vi "Receptor.vi"() -> ()   [LabVIEW 2012]
uses:
  VariavelGlobalTDD.vi
panel:
  out "x = y?":bool caption="Se TDD on > Teste Passou?"
  in  "Boolean":bool caption="TDD"
  in  "stop 2":bool
  out "Dado Recebido:":string
  # "Rodar este VI antes de rodar Emissor.vi."
  # "1- Escolher TDD on ou off no switch;\n2- Rodar este VI;"
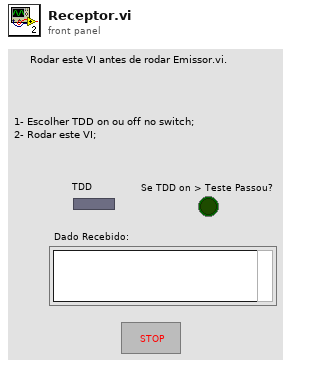
[diagram p1: front panel]
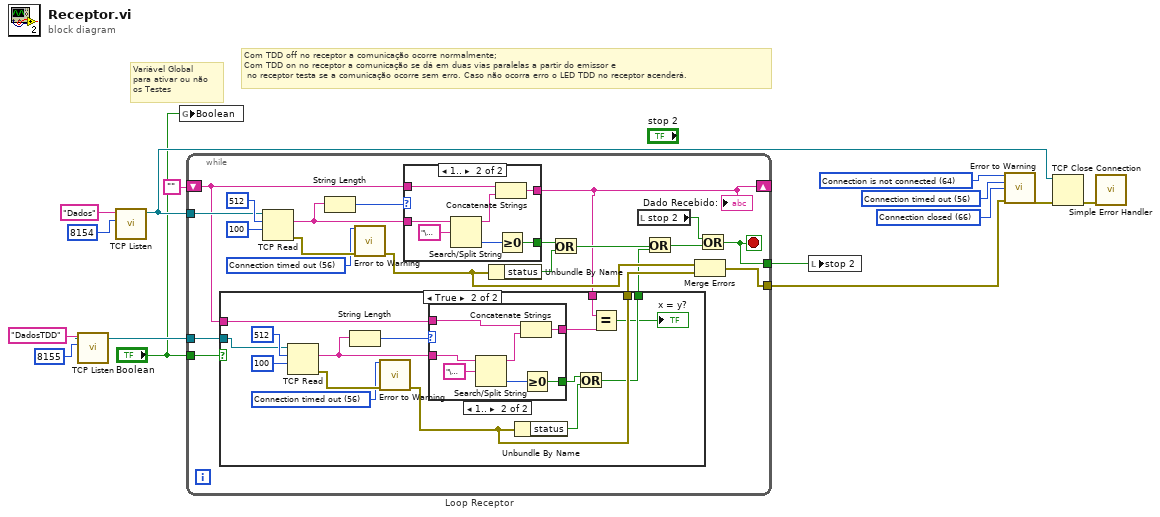
[diagram p0: block diagram]
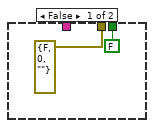
[diagram p2: hidden frame]
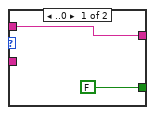
[diagram p3: hidden frame]
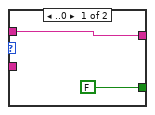
[diagram p4: hidden frame]
diagram:
  w8 = 56 items=["No Error", "Argument Error", "Memory Full", "Out of Zone", "End of File", "File Already Open", "Generic File IO Error", "File Not Found", "File Permission Error", "Disk Full", "Duplicate Path", "Too Many Files Open", "Not Enabled", "Resource File Not Found", "Cannot Add Resource", "Resource Not Found", "Image Not Found", "Image Memory Error", "Pen Does Not Exist", "Config Bad Type", "Config Token Not Found", "Config Parse Error", "Config Memory Error", "Bad External Code Format", "Bad External Code Offset", "External Code Not Present", "Null Window", "Destroy Window Mixup", "Null Menu", "Print Aborted", "Bad Print Record", "Print Driver Error", "Windows Error During Print", "Memory Error During Print", "Print Dialog Error", "Generic Print Error", "Invalid Device Refnum", "Device Not Found", "Device Parameter Error", "Device Unit Error", "Can't Open Device", "Device Call Aborted", "Generic Error", "Cancelled By User", "Object ID Too Low", "Object ID Too High", "Object Not In Heap", "Unknown Heap", "Bad DefProc ID", "DefProc Not In Table", "Message Out Of Range", "Null Method", "Unknown Message", "Manager Call Not Supported", "Bad address", "Connection In progress", "Connection timed out", "Connection is already in progress", "Network attribute not supported", "Network error", "Address in use", "System out of memory", "Connection aborted", "Connection refused", "Connection is not connected", "Connection is already connected", "Connection closed", "Initialize error (interapplication manager)", "Bad occurrence", "Wait on unbound occurrence handler", "Occurrence queue overflow", "Bad path", "Semaphore not signaled", "Unrecognized type (interapplication manager)"] ("2nd Error to Convert")
  w9 = 66 items=["No Error", "Argument Error", "Memory Full", "Out of Zone", "End of File", "File Already Open", "Generic File IO Error", "File Not Found", "File Permission Error", "Disk Full", "Duplicate Path", "Too Many Files Open", "Not Enabled", "Resource File Not Found", "Cannot Add Resource", "Resource Not Found", "Image Not Found", "Image Memory Error", "Pen Does Not Exist", "Config Bad Type", "Config Token Not Found", "Config Parse Error", "Config Memory Error", "Bad External Code Format", "Bad External Code Offset", "External Code Not Present", "Null Window", "Destroy Window Mixup", "Null Menu", "Print Aborted", "Bad Print Record", "Print Driver Error", "Windows Error During Print", "Memory Error During Print", "Print Dialog Error", "Generic Print Error", "Invalid Device Refnum", "Device Not Found", "Device Parameter Error", "Device Unit Error", "Can't Open Device", "Device Call Aborted", "Generic Error", "Cancelled By User", "Object ID Too Low", "Object ID Too High", "Object Not In Heap", "Unknown Heap", "Bad DefProc ID", "DefProc Not In Table", "Message Out Of Range", "Null Method", "Unknown Message", "Manager Call Not Supported", "Bad address", "Connection In progress", "Connection timed out", "Connection is already in progress", "Network attribute not supported", "Network error", "Address in use", "System out of memory", "Connection aborted", "Connection refused", "Connection is not connected", "Connection is already connected", "Connection closed", "Initialize error (interapplication manager)", "Bad occurrence", "Wait on unbound occurrence handler", "Occurrence queue overflow", "Bad path", "Semaphore not signaled", "Unrecognized type (interapplication manager)"] ("3rd Error to Convert")
  w10 = 64 items=["No Error", "Argument Error", "Memory Full", "Out of Zone", "End of File", "File Already Open", "Generic File IO Error", "File Not Found", "File Permission Error", "Disk Full", "Duplicate Path", "Too Many Files Open", "Not Enabled", "Resource File Not Found", "Cannot Add Resource", "Resource Not Found", "Image Not Found", "Image Memory Error", "Pen Does Not Exist", "Config Bad Type", "Config Token Not Found", "Config Parse Error", "Config Memory Error", "Bad External Code Format", "Bad External Code Offset", "External Code Not Present", "Null Window", "Destroy Window Mixup", "Null Menu", "Print Aborted", "Bad Print Record", "Print Driver Error", "Windows Error During Print", "Memory Error During Print", "Print Dialog Error", "Generic Print Error", "Invalid Device Refnum", "Device Not Found", "Device Parameter Error", "Device Unit Error", "Can't Open Device", "Device Call Aborted", "Generic Error", "Cancelled By User", "Object ID Too Low", "Object ID Too High", "Object Not In Heap", "Unknown Heap", "Bad DefProc ID", "DefProc Not In Table", "Message Out Of Range", "Null Method", "Unknown Message", "Manager Call Not Supported", "Bad address", "Connection In progress", "Connection timed out", "Connection is already in progress", "Network attribute not supported", "Network error", "Address in use", "System out of memory", "Connection aborted", "Connection refused", "Connection is not connected", "Connection is already connected", "Connection closed", "Initialize error (interapplication manager)", "Bad occurrence", "Wait on unbound occurrence handler", "Occurrence queue overflow", "Bad path", "Semaphore not signaled", "Unrecognized type (interapplication manager)"] ("1st Error to Convert")
  # "Variável Global\npara ativar ou não\nos Testes"
  # "Com TDD off no receptor a comunicação ocorre normalmente;\nCom TDD on no receptor a comunicação se dá em duas vias paralelas a partir do emissor e\n no receptor testa se a comunicação ocorre sem erro. Caso não ocorra erro o LED TDD no receptor acenderá."
  n1 = call <vilib>:"TCP Listen.vi"("port"=u16 8155, "service name"="DadosTDD" ("address")) -> ("connection ID"=w2:refnum<k5>)  [unwired: 5 in, 4 out]
  n2 = call <vilib>:"TCP Listen.vi"("port"=u16 8154, "service name"="Dados" ("address")) -> ("connection ID"=w5:refnum<k5>)  [unwired: 5 in, 4 out]
  n3 = global write "VariavelGlobalTDD.vi" "Boolean"("Boolean") -> ()
  n4 = while "Loop Receptor" {
    shift-left: "" -> [w22]
    shift-right: [w16] -> _
    tunnel: [w33] -> w12
    tunnel: [w23] -> w7
    tunnel: w5 -> [w34]
    tunnel: w2 -> [w21]
    tunnel: "Boolean" -> [w20]
    stop <- w33 stop-if-true
    w28 = 56 items=["No Error", "Argument Error", "Memory Full", "Out of Zone", "End of File", "File Already Open", "Generic File IO Error", "File Not Found", "File Permission Error", "Disk Full", "Duplicate Path", "Too Many Files Open", "Not Enabled", "Resource File Not Found", "Cannot Add Resource", "Resource Not Found", "Image Not Found", "Image Memory Error", "Pen Does Not Exist", "Config Bad Type", "Config Token Not Found", "Config Parse Error", "Config Memory Error", "Bad External Code Format", "Bad External Code Offset", "External Code Not Present", "Null Window", "Destroy Window Mixup", "Null Menu", "Print Aborted", "Bad Print Record", "Print Driver Error", "Windows Error During Print", "Memory Error During Print", "Print Dialog Error", "Generic Print Error", "Invalid Device Refnum", "Device Not Found", "Device Parameter Error", "Device Unit Error", "Can't Open Device", "Device Call Aborted", "Generic Error", "Cancelled By User", "Object ID Too Low", "Object ID Too High", "Object Not In Heap", "Unknown Heap", "Bad DefProc ID", "DefProc Not In Table", "Message Out Of Range", "Null Method", "Unknown Message", "Manager Call Not Supported", "Bad address", "Connection In progress", "Connection timed out", "Connection is already in progress", "Network attribute not supported", "Network error", "Address in use", "System out of memory", "Connection aborted", "Connection refused", "Connection is not connected", "Connection is already connected", "Connection closed", "Initialize error (interapplication manager)", "Bad occurrence", "Wait on unbound occurrence handler", "Occurrence queue overflow", "Bad path", "Semaphore not signaled", "Unrecognized type (interapplication manager)"] ("1st Error to Convert")
    n5 = TCP Read(connection ID=w34, bytes to read=512, 9:100) -> (data out=w32:string, error out=w29:errorcluster)  [unwired: 2 in, 1 out]
    n6 = String Length(string=w32) -> (length=w36:i32)
    n7 = call <vilib>:"Error to Warning.vi"("1st Error to Convert"=w28, "error in"=w29) -> ("warning out"=w25:errorcluster)  [unwired: 13 in]
    n8 = case shown="1.." w36 {
      tunnel: w32 -> [_ w68]
      tunnel: w22 -> [w64 w71]
      tunnel: [w64 w70] -> w16
      tunnel: [FALSE w65] -> w31
      frame ..0 {
      }
      frame 1.. {
        n9 = Search/Split String(string=w68, search string/char (-)="\u0004") -> (substring before match=w67:string, offset of match=w66:i32)  [unwired: 1 in, 1 out]
        n10 = Concatenate Strings(w71, w67) -> (w70:string)
        n11 = Greater Or Equal To 0?(x=w66) -> (x >= 0?=w65:bool)
      }
    }
    "Dado Recebido:" <- w16
    n12 = case shown="True" w20 {
      tunnel: [errorcluster {"status"=FALSE, "code"=0, "source"=""} ("warning out") w45] -> w24
      tunnel: w22 -> [_ w42]
      tunnel: w21 -> [_ w44]
      tunnel: [FALSE w43] -> w19
      tunnel: w16 -> [_ w41]
      frame False {
      }
      frame True {
        w47 = 56 items=["No Error", "Argument Error", "Memory Full", "Out of Zone", "End of File", "File Already Open", "Generic File IO Error", "File Not Found", "File Permission Error", "Disk Full", "Duplicate Path", "Too Many Files Open", "Not Enabled", "Resource File Not Found", "Cannot Add Resource", "Resource Not Found", "Image Not Found", "Image Memory Error", "Pen Does Not Exist", "Config Bad Type", "Config Token Not Found", "Config Parse Error", "Config Memory Error", "Bad External Code Format", "Bad External Code Offset", "External Code Not Present", "Null Window", "Destroy Window Mixup", "Null Menu", "Print Aborted", "Bad Print Record", "Print Driver Error", "Windows Error During Print", "Memory Error During Print", "Print Dialog Error", "Generic Print Error", "Invalid Device Refnum", "Device Not Found", "Device Parameter Error", "Device Unit Error", "Can't Open Device", "Device Call Aborted", "Generic Error", "Cancelled By User", "Object ID Too Low", "Object ID Too High", "Object Not In Heap", "Unknown Heap", "Bad DefProc ID", "DefProc Not In Table", "Message Out Of Range", "Null Method", "Unknown Message", "Manager Call Not Supported", "Bad address", "Connection In progress", "Connection timed out", "Connection is already in progress", "Network attribute not supported", "Network error", "Address in use", "System out of memory", "Connection aborted", "Connection refused", "Connection is not connected", "Connection is already connected", "Connection closed", "Initialize error (interapplication manager)", "Bad occurrence", "Wait on unbound occurrence handler", "Occurrence queue overflow", "Bad path", "Semaphore not signaled", "Unrecognized type (interapplication manager)"] ("1st Error to Convert")
        n13 = TCP Read(connection ID=w44, bytes to read=512, 9:100) -> (data out=w51:string, error out=w48:errorcluster)  [unwired: 2 in, 1 out]
        n14 = String Length(string=w51) -> (length=w53:i32)
        n15 = call <vilib>:"Error to Warning.vi"("1st Error to Convert"=w47, "error in"=w48) -> ("warning out"=w45:errorcluster)  [unwired: 13 in]
        n16 = case shown="1.." w53 {
          tunnel: w51 -> [_ w59]
          tunnel: w42 -> [w55 w62]
          tunnel: [w55 w61] -> w40
          tunnel: [FALSE w56] -> w50
          frame ..0 {
          }
          frame 1.. {
            n17 = Search/Split String(string=w59, search string/char (-)="\u0004") -> (substring before match=w58:string, offset of match=w57:i32)  [unwired: 1 in, 1 out]
            n18 = Concatenate Strings(w62, w58) -> (w61:string)
            n19 = Greater Or Equal To 0?(x=w57) -> (x >= 0?=w56:bool)
          }
        }
        n20 = Unbundle By Name(w45) -> ("status"=w46:bool)
        n21 = Or(x=w50, y=w46) -> (x .or. y?=w43:bool)
        n22 = Equal?(x=w41, y=w40) -> (x = y?=→"x = y?":bool)
      }
    }
    n23 = Unbundle By Name(w25) -> ("status"=w27:bool)
    n24 = Or(x=w31, y=w27) -> (x .or. y?=w18:bool)
    n25 = local read "stop 2"() -> (w26:bool)
    n26 = Or(x=w18, y=w19) -> (x .or. y?=w17:bool)
    n27 = Merge Errors(w25, w24) -> (w23:errorcluster)
    n28 = Or(x=w26, y=w17) -> (x .or. y?=w33:bool)
  }
  n29 = local write "stop 2"(w12) -> ()
  n30 = call <vilib>:"Error to Warning.vi"("1st Error to Convert"=w10, "2nd Error to Convert"=w8, "3rd Error to Convert"=w9, "error in"=w7) -> ("warning out"=w6:errorcluster)  [unwired: 11 in]
  n31 = TCP Close Connection(connection ID=w5, error in (no error)=w6) -> (error out=w11:errorcluster)  [unwired: 1 in, 1 out]
  n32 = call <vilib>:"Simple Error Handler.vi"("error in (no error)"=w11) -> ()  [unwired: 4 in, 5 out]
